vi "DeviceFind.vi"(8 "error in (no error)":errorcluster caption="错误输入（无错误）") -> (0 "error out":errorcluster caption="错误输出", 1 "SNs":string[](array[string]), 2 "Descriptions":string[](array[string]), 3 "function return":i32, 5 "设备数量":u32)   [LabVIEW 2018]
doc: "Find all device and return count ,descripts and SNs"
uses:
  InstrumentsPlayground.lvlib
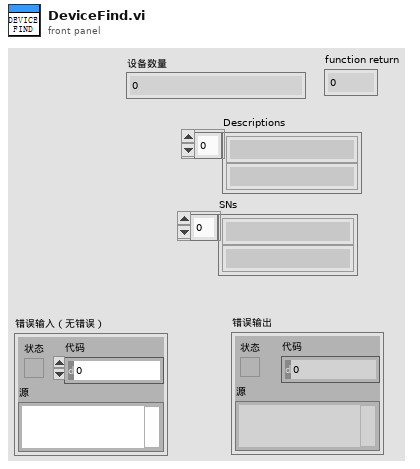
[diagram p1: front panel]
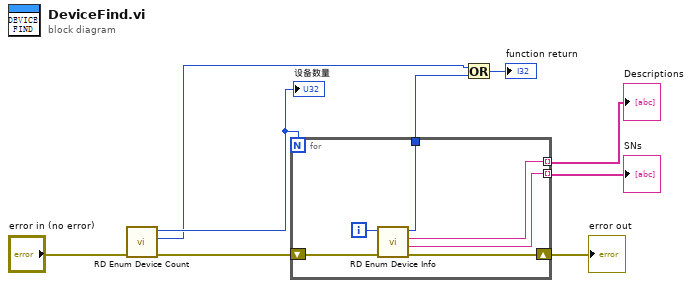
[diagram p0: block diagram]
diagram:
  n1 = call "RD Enum Device Count.vi"("error in (no error)"="error in (no error)") -> ("error out"=w6:errorcluster, "function return"=w4:i32, "count out"=w9:u32)  [unwired: 8 in]
  "设备数量" <- w9
  n2 = for {
    N: w9 -> [_]
    tunnel: [w14] -> w8 mode=indexing
    tunnel: [w13] -> w7 mode=indexing
    shift-right: [w11] -> w1
    shift-left: w6 -> [w12]
    tunnel: [w10] -> w5
    i -> [w15]
    n3 = call "RD Enum Device Info.vi"("error in (no error)"=w12, "i"=w15) -> ("error out"=w11:errorcluster, "SerialNumber out"=w13:string, "Description out"=w14:string, "function return"=w10:i32)  [unwired: 5 in, 1 out]
  }
  "error out" <- w1
  "Descriptions" <- w8
  "SNs" <- w7
  n4 = Or(x=w4, y=w5) -> (x .or. y?=→"function return":i32)
